vi "TC-Version.vi"() -> (0 "TC Version":string)   [LabVIEW 2019]
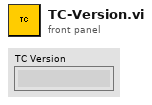
[diagram p1: front panel]
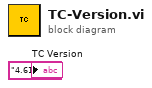
[diagram p0: block diagram]
diagram:
  "TC Version" <- "4.61.7.12"
